vi "VI Linearisierung v2.vi"() -> ()   [LabVIEW 2020, in "Linearisierung v2.lvlib"] (continued)
                # "running erst setzen, wenn der Gasteiler bereits aus Beenden raus ist ,\nsonst triggert er im Timeout schon wieder ... !!!"
                n1604 = case shown="Kein Fehler" w2827 {
                  frame No Error {
                    n1605 = call "FGV SpanEinstellungen.vi"("Aktion"=Aktion_FGV_SpanEinstellungen."lesen") -> ("automatisch out"=w2832:T20)  [unwired: 6 in, 4 out]
                    n1606 = call "FGV Daten Abholung uebergeben.vi"("Aktion"=Aktion_FGV_Daten_Abholung_uebergebenctl."lesen") -> ("Beendet"=w2830:bool)  [unwired: 10 in, 4 out]
                    n1607 = call "FGV Gasteiler.vi"("Aktionen"=Aktionen_FGV_Gasteiler_Daten."lesen") -> ("Aufzeichnung Start"=w2828:bool)  [unwired: 11 in, 7 out]
                    n1608 = case shown="True" w2832 {
                      tunnel: w2830 -> [_ _]
                      tunnel: w2828 -> [_ _]
                      frame False {
                        # "brauchen wir hier auch !"
                        n1609 = call "FGV Spans abarbeiten.vi"("running"=TRUE, "Aktion"=Aktion_FGV_Spans_abarbeiten."running") -> ()  [unwired: 4 in, 6 out]
                      }
                      frame True {
                        # "für Start und Next erst hier"
                        n1610 = call "FGV Spans abarbeiten.vi"("running"=TRUE, "Aktion"=Aktion_FGV_Spans_abarbeiten."running") -> ()  [unwired: 4 in, 6 out]
                      }
                    }
                  }
                  frame Error {
                  }
                }
              }
              frame #5 {
                w2838 = T1 FALSE ("EPA Filename override")
                # "#LinV2_auto_singleSave"
                # "#RickQuickTest_Features"
                n1611 = call "FGV SpanEinstellungen.vi"("Aktion"=Aktion_FGV_SpanEinstellungen."lesen") -> ("Punkte umkehren und PDF Optionen Cluster"=w2840:T109)  [unwired: 6 in, 4 out]
                n1612 = Unbundle By Name(w2840) -> ("PDF Optionen.Graphik für Messwerte"=w2839:bool)
                n1613 = case shown="True" w2839 {
                  frame False {
                  }
                  frame True {
                    n1614 = call "LIN Graph.vi"() -> ()  [unwired: 12 in]
                  }
                }
                n1615 = local write "EPA Filename override"(w2838) -> ()
                n1616 = local write "LIN Filename override"(w2838) -> ()
              }
            }
          }
        }
        n1617 = local write "STARTEN"(w2640) -> ()
      }
      event Value Change {
        # "#Option10xSpanAuto"
        n1618 = event-data() -> ()  [unwired: 1 in, 1 out]
        n1619 = call "FGV Stoerungen sammeln und auswerten.vi"("Aktion"=Aktion_FGV_Stoerungen_sammeln_und_auswerten."lesen") -> ("Error"=w2848:bool)  [unwired: 12 in, 6 out]
        n1620 = disable-structure shown="Aktiviert" {
          frame Disabled {
            n1621 = call "FGV Spans abarbeiten.vi"("Aktion"=Aktion_FGV_Spans_abarbeiten."idle") -> ("error out"=w2862:errorcluster)  [unwired: 5 in, 5 out]
            n1622 = call "FGV SPAN Verriegelung.vi"("aktion"=Aktion_FGV_SPAN_Verriegelung."unlock", "error in (no error)"=w2862) -> ("error out"=w2861:errorcluster)  [unwired: 7 in, 2 out]
            n1623 = call "FGV Post Processing.vi"("Aktion"=Aktion_FGV_Post_Processing."reset", "error in (no error)"=w2861) -> ()  [unwired: 6 in, 4 out]
          }
          frame Enabled {
            # "#ALIN_Cancel_Save"
            n1624 = control-ref of="Speichern LIN"() -> (w2872:refnum<vi>)
            n1625 = call "FGV Spans abarbeiten.vi"("Aktion"=Aktion_FGV_Spans_abarbeiten."lesen") -> ("active SPAN Idx out"=w2868:i32)  [unwired: 5 in, 5 out]
            n1626 = call "FGV SpanEinstellungen.vi"("Aktion"=Aktion_FGV_SpanEinstellungen."lesen") -> ("SpanInletClusterArray out"=w2869:T19[])  [unwired: 6 in, 4 out]
            n1627 = call "get first active SPAN.vi"("SpanInletClusterArray in"=w2869) -> ("Index first active SPAN"=w2867:i32, "SpanInletClusterArray out"=w2865:T19[])  [unwired: 8 in, 1 out]
            n1628 = Greater?(x=w2868, y=w2867) -> (0:w2866:bool)
            n1629 = case shown="False" w2866 {
              tunnel: w2872 -> [_ w2883]
              tunnel: w2865 -> [_ w2880]
              frame False {
                # "nothing to save ..."
                n1630 = call "FGV Spans abarbeiten.vi"("Aktion"=Aktion_FGV_Spans_abarbeiten."idle") -> ("error out"=w2875:errorcluster)  [unwired: 5 in, 5 out]
                n1631 = call "FGV SPAN Verriegelung.vi"("aktion"=Aktion_FGV_SPAN_Verriegelung."unlock", "error in (no error)"=w2875) -> ("error out"=w2874:errorcluster)  [unwired: 7 in, 2 out]
                n1632 = call "FGV Post Processing.vi"("Aktion"=Aktion_FGV_Post_Processing."reset", "error in (no error)"=w2874) -> ()  [unwired: 6 in, 4 out]
              }
              frame True {
                n1633 = call "FGV Spans abarbeiten.vi"("Aktion"=Aktion_FGV_Spans_abarbeiten."abort") -> ("error out"=w2879:errorcluster)  [unwired: 5 in, 5 out]
                n1634 = call "FGV Post Processing.vi"("Aktion"=Aktion_FGV_Post_Processing."abort", "error in (no error)"=w2879, "SpanInletClusterArray in"=w2880) -> ("error out"=w2878:errorcluster)  [unwired: 5 in, 3 out]
                n1635 = call "FGV Spans abarbeiten.vi"("running"=FALSE, "Aktion"=Aktion_FGV_Spans_abarbeiten."running", "error in (no error)"=w2878) -> ("error out"=w2884:errorcluster)  [unwired: 3 in, 5 out]
                n1636 = property on="Eigenschaftsknoten" class="Bool. (strikt)"(reference=w2883, error in=w2884, "Val(Sgnl)"=T4 TRUE ("Wert (signalisierend)")) -> (error out=w2887:errorcluster)  [unwired: 1 out]
                n1637 = call <vilib>:"Clear Errors.vi"("error in (no error)"=w2887) -> ()  [unwired: 5 in, 2 out]
              }
            }
          }
        }
        n1638 = property class="Bool."(reference=w2843, "DisabledEnum"=T66."Disabled and Grayed Out" ("Deaktiviert")) -> (error out=w2845:errorcluster)  [unwired: 1 in, 1 out]
        n1639 = call "FGV Gasteiler.vi"("Aufzeichnung Start"=FALSE ("STARTEN"), "Aktionen"=Aktionen_FGV_Gasteiler_Daten."Aufzeichnung Start") -> ()  [unwired: 10 in, 8 out]
        n1640 = And(x=w2848, y="ABBRECHEN") -> (x .and. y?=w2850:T4)
        n1641 = call <vilib>:"Clear Errors.vi"("error in (no error)"=w2845) -> ()  [unwired: 5 in, 2 out]
        n1642 = call "FGV Stoerungen sammeln und auswerten.vi"("Abbrechen"=w2850, "Aktion"=Aktion_FGV_Stoerungen_sammeln_und_auswerten."abbrechen") -> ("error out"=w2853:errorcluster)  [unwired: 11 in, 6 out]
        n1643 = property on="FORTSETZEN" class="Bool."(error in=w2853, "Visible"=FALSE ("Sichtbar")) -> (error out=w2855:errorcluster)  [unwired: 1 in, 1 out]
        n1644 = call <vilib>:"Clear Errors.vi"("error in (no error)"=w2855) -> ("error out"=w2851:errorcluster)  [unwired: 5 in, 1 out]
        n1645 = call "FGV Stoerungen sammeln und auswerten.vi"("error in (no error)"=w2851, "Aktion"=Aktion_FGV_Stoerungen_sammeln_und_auswerten."reset error") -> ()  [unwired: 11 in, 7 out]
      }
      event "post processing": Value Change {
        # "#LIN_only_saved_Polynoms"
        n1646 = event-data() -> ("OldVal"=w2891:u16)  [unwired: 1 in, 5 out]
        n1647 = Greater Than 0?(x="post processing") -> (x > 0?=w2890:bool)
        n1648 = Decrement(x="post processing") -> (x-1=w2889:u16)
        n1649 = case shown="False" w2890 {
          tunnel: w2889 -> [_ w2910]
          tunnel: w2893 -> [_ w2911]
          tunnel: w2891 -> [w2897 w2907]
          frame False {
            n1650 = call "FGV SPAN Verriegelung.vi"("aktion"=Aktion_FGV_SPAN_Verriegelung."lesen") -> ("Flags Cluster"=w2900:T188)  [unwired: 8 in, 2 out]
            n1651 = local write "post processing"(w2897) -> ()
            n1652 = Unbundle By Name(w2900) -> ("Postprocessing PDF"=w2898:bool)
            n1653 = case shown="True" w2898 {
              frame False {
              }
              frame True {
                n1654 = local write "post processing PDFs"(T4 FALSE ("post processing PDFs")) -> ()
                n1655 = call "FGV SPAN Verriegelung.vi"("aktion"=Aktion_FGV_SPAN_Verriegelung."Reset Postprocessing PDF") -> ()  [unwired: 8 in, 3 out]
              }
            }
          }
          frame True {
            n1656 = Decrement(x=w2907) -> (x-1=w2906:u16)
            n1657 = call "FGV Post Processing.vi"("Aktion"=Aktion_FGV_Post_Processing."lesen") -> ("filenemas Cluster Array"=w2917:T211, "Index active SPANs"=w2909:i32[])  [unwired: 7 in, 2 out]
            n1658 = call "FGV SPAN Verriegelung.vi"("aktion"=Aktion_FGV_SPAN_Verriegelung."lesen") -> ("Flags Cluster"=w2905:T188)  [unwired: 8 in, 2 out]
            n1659 = Unbundle By Name(w2905) -> ("Postprocessing PDF"=w2903:bool)
            n1660 = Index Array(array=w2909, index=w2910) -> (element=w2913:i32)
            n1661 = Index Array(array=w2917, index=w2910) -> (element=w2916:T212)
            n1662 = Index Array(array=w2909, index=w2906) -> (element=w2908:i32)
            n1663 = Unbundle By Name(w2916) -> ("active SPAN Idx"=w2912:i32, "Pfad .LIN Datei"=w2915:T9)
            n1664 = Equal?(x=w2913, y=w2912) -> (x = y?=w2914:bool)
            n1665 = case shown="True" w2914 {
              tunnel: w2915 -> [_ w2954]
              tunnel: w2913 -> [w2924 w2930]
              tunnel: w2912 -> [w2922 _]
              tunnel: w2911 -> [_ w2952]
              tunnel: w2910 -> [_ w2946]
              tunnel: w2908 -> [_ w2942]
              tunnel: w2906 -> [_ w2934]
              tunnel: w2903 -> [_ w2927]
              tunnel: w2903 -> [_ w2926]
              frame False {
                n1666 = Number To Decimal String(number=w2924) -> (decimal integer string=w2923:string)  [unwired: 1 in]
                n1667 = Number To Decimal String(number=w2922) -> (decimal integer string=w2921:string)  [unwired: 1 in]
                n1668 = Concatenate Strings("internal Error: active SPAN ", w2923, " <> " ("String"), w2921) -> (w2919:string)
                n1669 = One Button Dialog(message=w2919) -> ()  [unwired: 1 in, 1 out]
              }
              frame True {
                w2945 = 0  # Component Idx
                # "#Lin_Load_Polynom_Question"
                n1670 = case shown="False" w2927 {
                  tunnel: w2942 -> [w2962 _]
                  tunnel: [w2961 _] -> w2935
                  tunnel: w2934 -> [w2960 _]
                  frame False {
                    n1671 = call "PostProcessing_LIN_speichern.vi"("Index active SPAN"=w2962, "reprocessing index for filname"=w2960) -> ("Fehler (Ausgang)"=w2961:errorcluster)  [unwired: 9 in]
                  }
                  frame True {
                  }
                }
                n1672 = call "Set SPAN Komponentauswahl in Protokolldaten.vi"("error in (no error)"=w2935, "index of element"=w2930) -> ("error out"=w2937:errorcluster, "original Lin-Polynom"=w2936:T119)  [unwired: 8 in]
                n1673 = Bundle("Index active SPAN"=w2930, "Component Idx"=w2945, w2946) -> (w2947:T213)  [unwired: 1 in]
                n1674 = call "FGV SpanEinstellungen.vi"("Aktion"=Aktion_FGV_SpanEinstellungen."lesen") -> ("SpanInletClusterArray out"=w2931:T19[])  [unwired: 6 in, 4 out]
                n1675 = call "LinDaten speichern und laden.vi"("Aktion"=enum16{"speichern", "laden"}."speichern", "error in (no error)"=w2937) -> ("error out"=w2955:errorcluster, "LIN Protokoll Daten"=w2943:T119, "Setup Daten-Cluster"=w2940:T204, "Settings Cluster"=w2941:T206)  [unwired: 3 in, 3 out]
                n1676 = Index Array(array=w2931, index=w2930) -> (element=w2933:T19)
                n1677 = Unbundle By Name(w2943) -> ("Messgerät"=w2944:string)
                n1678 = Unbundle By Name(w2933) -> ("Max Fehler"=w2928:sgl)
                n1679 = call "LinDaten speichern und laden.vi"("Aktion"=enum16{"speichern", "laden"}."laden", "error in (no error)"=w2955, "Analysator"=w2944, "selected path"=w2954) -> ("error out"=w2957:errorcluster, "LIN Protokoll Daten"=w2948:T119, "MessDaten Array"=w2949:string[][][], "Ident Cluster"=w2958:T205, "Setup Daten-Cluster"=w2938:T204, "Settings Cluster"=w2939:T206)  [unwired: 1 in, 1 out]
                n1680 = Bundle By Name(cluster=w2948, "F_max gefordert (%)"=w2928) -> (w2929:T119)
                n1681 = call "LIN Laden Errors.vi"("Fehler (Eingang, kein Fehler)"=w2957, "Ident Cluster"=w2958) -> ("Error orccured"=w2953:bool, "LIN Loading Error Description Array"=w2951:T207, "LIN Loading Errors Array"=w2950:string[])  [unwired: 5 in, 2 out]
                n1682 = case shown="False" w2953 {
                  tunnel: w2952 -> [_ w2993]
                  tunnel: w2951 -> [_ _]
                  tunnel: w2950 -> [_ w2986]
                  tunnel: w2949 -> [w2980 _]
                  tunnel: w2929 -> [w2970 _]
                  tunnel: w2947 -> [w2976 _]
                  tunnel: w2941 -> [w2974 _]
                  tunnel: w2940 -> [w2973 _]
                  tunnel: w2939 -> [w2972 _]
                  tunnel: w2938 -> [w2971 _]
                  tunnel: w2936 -> [_ w2987]
                  tunnel: w2930 -> [w2966 _]
                  tunnel: w2926 -> [w2963 _]
                  frame False {
                    n1683 = call "Lin Daten aufarbeiten.vi"("Lin-Polynom"=w2970, "Aktionen"=Aktion_Lin_Daten_aufarbeiten."Protkolldaten") -> ("Lin-Polynom"=w2968:T119, "error out"=w2969:errorcluster)  [unwired: 15 in, 9 out]
                    n1684 = call "Lin Daten aufarbeiten.vi"("error in (no error)"=w2969, "TabellenArray"=w2980, "Aktionen"=Aktion_Lin_Daten_aufarbeiten."Nachbehandlung laden") -> ("error out"=w2967:errorcluster)  [unwired: 14 in, 10 out]
                    n1685 = call "LIN Laden Polynom setzen.vi"("Span Iindex"=w2966, "Settings Cluster old"=w2974, "Setup Daten-Cluster old"=w2973, "error in (no error)"=w2967, "LIN Protokoll Daten"=w2968, "Setup Daten-Cluster new"=w2971, "Settings Cluster new"=w2972) -> ("error out"=w2965:errorcluster)  [unwired: 4 in]
                    n1686 = call "FGV Post Processing.vi"("Aktion"=Aktion_FGV_Post_Processing."active", "error in (no error)"=w2965, "active Index Cluster in"=w2976) -> ("error out"=w2977:errorcluster)  [unwired: 5 in, 3 out]
                    n1687 = property on="Gasnummer Generieren" class="DigWert (strikt)"(error in=w2977, "Val(Sgnl)"=T49 1 ("Wert (signalisierend)")) -> (error out=w2964:errorcluster)  [unwired: 1 in, 1 out]
                    n1688 = case shown="True" w2963 {
                      tunnel: w2964 -> [_ w2982]
                      frame False {
                      }
                      frame True {
                        n1689 = property on="Speichern LIN" class="Bool. (strikt)"(error in=w2982, "Val(Sgnl)"=T4 TRUE ("Wert (signalisierend)")) -> (error out=w2984:errorcluster)  [unwired: 1 in, 1 out]
                        n1690 = call <vilib>:"Clear Errors.vi"("error in (no error)"=w2984) -> ()  [unwired: 5 in, 2 out]
                      }
                    }
                  }
                  frame True {
                    # "reset"
                    n1691 = call "Lin Daten aufarbeiten.vi"("Lin-Polynom"=w2987, "Aktionen"=Aktion_Lin_Daten_aufarbeiten."Protkolldaten") -> ()  [unwired: 15 in, 11 out]
                    n1692 = call "Texte in VIs uebersetzen.vi"("Sprachliste"=w2993, "String-Array zum Übersetzen"=w2986, "String zum Übersetzen"="Loading LIN Date does not fit actual Setup!") -> ("String-Array zum Übersetzen"=w2985:string[], "String zum Übersetzen"=w2994:string)  [unwired: 8 in, 3 out]
                    n1693 = call <vilib>:"1D String Array to Delimited String.vi"("delimiter"=",", "string array"=w2985) -> ("delimited string"=w2989:string)  [unwired: 9 in]
                    n1694 = Concatenate Strings(w2994, " - " ("String"), w2989) -> (w2992:string)
                    n1695 = One Button Dialog(message=w2992) -> ()  [unwired: 1 in, 1 out]
                  }
                }
              }
            }
          }
        }
      }
      event Value Change {
        n1696 = event-data() -> ()  [unwired: 1 in, 6 out]
        n1697 = call "FGV SPAN Verriegelung.vi"("aktion"=Aktion_FGV_SPAN_Verriegelung."lesen") -> ("Flags Cluster"=w2997:T188)  [unwired: 8 in, 2 out]
        n1698 = Unbundle By Name(w2997) -> ("Postprocessing PDF"=w2996:bool)
        n1699 = case shown="False" w2996 {
          tunnel: w2999 -> [w3004 _]
          frame False {
            n1700 = call "Texte in VIs uebersetzen.vi"("Sprachliste"=w3004, "String zum Übersetzen"="Alle PDF vom Postprocessing speichern?" ("Nachricht")) -> ("String zum Übersetzen"=w3010:string)  [unwired: 9 in, 4 out]
            n1701 = call "Texte in VIs uebersetzen.vi"("Sprachliste"=w3004, "String zum Übersetzen"="Ja" ("Text für T-Schaltfläche (\"OK\")")) -> ("String zum Übersetzen"=w3009:string)  [unwired: 9 in, 4 out]
            n1702 = call "Texte in VIs uebersetzen.vi"("Sprachliste"=w3004, "String zum Übersetzen"="Nein" ("Text für F-Schaltfläche (\"Abbrechen\")")) -> ("String zum Übersetzen"=w3008:string)  [unwired: 9 in, 4 out]
            n1703 = Two Button Dialog(message=w3010, 1:w3008, 2:w3009) -> (T button?=w3003:bool)
            n1704 = case shown="True" w3003 {
              frame False {
              }
              frame True {
                w3011 = FALSE
                # "#LinV2_auto_singleSave"
                # "letzte Änderung beim ersten Aufruf speichern\nruft signalisierend Postprocessing Span Auswahl auf ..."
                n1705 = local read "post processing"() -> (w3019:u16)
                n1706 = call "FGV Post Processing.vi"("Aktion"=Aktion_FGV_Post_Processing."lesen") -> ("Index active SPANs"=w3018:i32[])  [unwired: 7 in, 3 out]
                n1707 = Decrement(x=w3019) -> (x-1=w3012:u16)
                n1708 = Index Array(array=w3018, index=w3012) -> (element=w3020:i32)
                n1709 = call "PostProcessing_LIN_speichern.vi"("Index active SPAN"=w3020, "reprocessing index for filname"=w3012) -> ("Fehler (Ausgang)"=w3013:errorcluster)  [unwired: 9 in]
                n1710 = call "FGV SPAN Verriegelung.vi"("aktion"=Aktion_FGV_SPAN_Verriegelung."Set Postprocessing PDF", "error in (no error)"=w3013) -> ("error out"=w3016:errorcluster)  [unwired: 7 in, 2 out]
                n1711 = local write "EPA Filename override"(w3011) -> ()
                n1712 = local write "LIN Filename override"(w3011) -> ()
                n1713 = call "FGV Post Processing.vi"("Aktion"=Aktion_FGV_Post_Processing."first", "error in (no error)"=w3016) -> ()  [unwired: 6 in, 4 out]
              }
            }
          }
          frame True {
            # "läuft schon"
            n1714 = local write "post processing PDFs"(T4 FALSE ("post processing PDFs")) -> ()
          }
        }
      }
      event Value Change {
        n1715 = event-data() -> ()  [unwired: 1 in, 1 out]
        n1716 = local write "post processing done"(T4 FALSE ("post processing done")) -> ()
        n1717 = call "Texte in VIs uebersetzen.vi"("Sprachliste"=w3024, "String zum Übersetzen"="Fertig mit Postprocessing?\nFreigabe löscht die gesammelten Daten!" ("Nachricht")) -> ("String zum Übersetzen"=w3026:string)  [unwired: 9 in, 4 out]
        n1718 = call "Texte in VIs uebersetzen.vi"("Sprachliste"=w3024, "String zum Übersetzen"="Ja" ("Text für T-Schaltfläche (\"OK\")")) -> ("String zum Übersetzen"=w3027:string)  [unwired: 9 in, 4 out]
        n1719 = call "Texte in VIs uebersetzen.vi"("Sprachliste"=w3024, "String zum Übersetzen"="Nein" ("Text für F-Schaltfläche (\"Abbrechen\")")) -> ("String zum Übersetzen"=w3028:string)  [unwired: 9 in, 4 out]
        n1720 = Two Button Dialog(message=w3026, 1:w3028, 2:w3027) -> (T button?=w3025:bool)
        n1721 = case shown="True" w3025 {
          frame False {
          }
          frame True {
            n1722 = call "FGV Post Processing.vi"("Aktion"=Aktion_FGV_Post_Processing."reset") -> ("error out"=w3034:errorcluster)  [unwired: 7 in, 3 out]
            n1723 = call "FGV SPAN Verriegelung.vi"("aktion"=Aktion_FGV_SPAN_Verriegelung."unlock", "error in (no error)"=w3034) -> ()  [unwired: 7 in, 3 out]
          }
        }
      }
      event Value Change {
        # "#LIN_only_saved_Polynoms"
        # "#PDF_manu_MG"
        n1724 = event-data() -> ()  [unwired: 1 in, 1 out]
        n1725 = call "Komponentenausgabe.vi"() -> ("Gaskomponente"=w3051:T7)  [unwired: 8 in, 3 out]
        n1726 = local read "Gasnummer LIN"() -> (w3042:T49)
        n1727 = call "Lin Daten aufarbeiten.vi"("Index (Seite)"=w3051, "Polynom-Ordnung"="Polynom-Ordnung", "Aktionen"=Aktion_Lin_Daten_aufarbeiten."Lin auswerten") -> ("Index (Seite) out"=w3044:i32, "error out"=w3053:errorcluster)  [unwired: 14 in, 9 out]
        n1728 = call "aktueller SPAN und Komponent Index.vi"() -> ("akt SPAN out"=w3039:i32)  [unwired: 7 in, 4 out]
        n1729 = Decrement(x=w3042) -> (x-1=w3038:T49)
        n1730 = Bundle("akt SPAN out"=w3039, w3038) -> (w3037:cluster{"akt SPAN out":i32, T49})  [unwired: 1 in]
        n1731 = call "Lin Daten aufarbeiten.vi"("Index (Seite)"=w3044, "error in (no error)"=w3053, "Aktionen"=Aktion_Lin_Daten_aufarbeiten."lesen") -> ("Eingabetabelle"=w3052:T54, "Lin-Polynom"=w3049:T119)  [unwired: 14 in, 9 out]
        n1732 = call "LIN Polynom Ordnung je Komponente für Protokoll.vi"("Aktion"=Aktion_LIN_Polynom_Ordnung_je_Komponente_für_Protokoll."schreiben viewonly", "Polynom-Ordnung view only"="Polynom-Ordnung", "Index in"=w3037) -> ()  [unwired: 2 in, 7 out]
        n1733 = Unbundle By Name(w3049) -> ("Polynomkoeff."=w3048:dbl[])
        n1734 = call "LinTabelle zusammenbauen.vi"("Eingabetabelle"=w3052) -> ("XY-Graph"=w3050:cluster{dbl[], dbl[]}[], "LIN Ausgabetabelle"=w3056:string[][])  [unwired: 7 in, 2 out]
        n1735 = local write "LIN Ausgabetabelle"(w3056) -> ()
        n1736 = local write "XY-Graph LIN"(w3050) -> ()
        n1737 = Array To Cluster(array=w3048) -> (cluster=→"LIN Polynomkoeffizienten":T185)
      }
      event Value Change {
        n1738 = event-data() -> ()  [unwired: 1 in, 1 out]
        n1739 = stacked-sequence {
          seq-local: [_ w3072 _ _] -> [_ _ w3095 _]
          seq-local: [_ w3071 _ _] -> [_ _ w3094 _]
          seq-local: [_ w3070 _ _] -> [_ _ w3096 _]
          seq-local: [_ _ w3088 _] -> [_ _ _ w3115]
          tunnel: w3060 -> [_ _ w3087 w3118]
          frame #0 {
            # "#LIN_only_saved_Polynoms"
            n1740 = call "Lin Daten aufarbeiten.vi"("Aktionen"=Aktion_Lin_Daten_aufarbeiten."lesen") -> ("Lin-Polynom"=w3068:T119)  [unwired: 16 in, 10 out]
            n1741 = Unbundle By Name(w3068) -> ("Polynomkoeff."=w3064:dbl[])
            n1742 = call "Komponentenausgabe.vi"() -> ("Gaskomponente"=w3061:T7)  [unwired: 8 in, 3 out]
            n1743 = call "Polynom Daten speichern.vi"("Aktionen"=Aktionen_Polynom_Daten_speichern."schreiben", "Einzelnes Polynom"=w3064, "Komponente"=w3061) -> ("Aktiv"=w3067:bool[])  [unwired: 3 in, 5 out]
            n1744 = call "Polynom Daten speichern.vi"("Aktionen"=Aktionen_Polynom_Daten_speichern."aktivieren", "Aktiv"=w3067, "Komponente"=w3061) -> ("Aktiv"=w3062:bool[])  [unwired: 3 in, 5 out]
            n1745 = call "Polynom Daten speichern.vi"("Aktionen"=Aktionen_Polynom_Daten_speichern."speichern", "Aktiv"=w3062) -> ()  [unwired: 4 in, 6 out]
          }
          frame #1 {
            # "#LIN_only_saved_Polynoms\nIstwerte mit neuem Polynom neu berechnen und anzeigen.\nEinstellungen speichern für Protokoll,\nin .LIN ebenfalls und wieder laden !\naktuell: aktuell + ---, 1...4\nautom.: automatisch + keine, 1...4\nmanuell: manuell + keine, 1...4\nraw: manuell + keine"
            n1746 = call "Komponentenausgabe.vi"() -> ("error out"=w3085:errorcluster, "Gaskomponente"=w3084:T7)  [unwired: 8 in, 2 out]
            n1747 = call "Lin Daten aufarbeiten.vi"("Index (Seite)"=w3084, "error in (no error)"=w3085, "Aktionen"=Aktion_Lin_Daten_aufarbeiten."LIN übernehmen") -> ("Index (Seite) out"=w3074:i32, "error out"=w3075:errorcluster)  [unwired: 14 in, 9 out]
            n1748 = call "aktueller SPAN und Komponent Index.vi"() -> ("akt SPAN out"=w3072:i32, "SpanInletClusterArray out"=w3070:T19[])  [unwired: 7 in, 3 out]
            n1749 = call "Lin Daten aufarbeiten.vi"("Index (Seite)"=w3074, "error in (no error)"=w3075, "Aktionen"=Aktion_Lin_Daten_aufarbeiten."lesen") -> ("Eingabetabelle"=w3077:T54, "error out"=w3076:errorcluster)  [unwired: 14 in, 9 out]
            n1750 = local read "Polynom-Ordnung"() -> (w3079:T55)
            n1751 = local read "Gasnummer LIN"() -> (w3086:T49)
            n1752 = call "LinTabelle zusammenbauen.vi"("error in (no error)"=w3076, "Eingabetabelle"=w3077) -> ("error out"=w3081:errorcluster, "LIN Ausgabetabelle"=w3082:string[][])  [unwired: 6 in, 2 out]
            n1753 = Decrement(x=w3086) -> (x-1=w3071:T49)
            n1754 = Bundle("akt SPAN out"=w3072, w3071) -> (w3073:cluster{"akt SPAN out":i32, T49})  [unwired: 1 in]
            n1755 = call "LIN Polynom Ordnung je Komponente für Protokoll.vi"("Aktion"=Aktion_LIN_Polynom_Ordnung_je_Komponente_für_Protokoll."schreiben", "error in (no error)"=w3081, "Index in"=w3073, "Polynom-Ordnung"=w3079) -> ()  [unwired: 1 in, 7 out]
            n1756 = local write "LIN Ausgabetabelle"(w3082) -> ()
          }
          frame #2 {
            # "Changes Flag setzen (vor der nächsten postprocess Auswahl dann .LIN speichern)\nKontrollieren ob in eine der Komponenten eines anderen SPAN die selbe ist,\ndann Warnung das kontrolliert werden soll, weil das dann automatisch auch so gerechnet wird beim Speichern wenn Done.\nBeim Laden der .LIN wird ein ungleiches Polynom erkannt und der Istwert neu berechnet (mit Hinweis) \nund die Polynomauswahl auf \"automatisch\" gesetzt."
            n1757 = call "get SPANs for same components in postprocessing.vi"("active Component Index"=w3094, "active SPAN Idx"=w3095, "SpanInletClusterArray in"=w3096) -> ("error out"=w3091:errorcluster, "active SPAN Idx out"=w3093:i32, "SPAN Index Array mit gleicher Komponente"=w3090:i32[], "found"=w3092:bool)  [unwired: 2 in, 3 out]
            n1758 = call "LIN Polynom Ordnung oder Aktiv Changes für Postprocessing.vi"("Aktion"=Aktion_LIN_Polynom_Ordnung_ode_Aktiv_Changes_für_Postprocessing."schreiben", "error in (no error)"=w3091, "active SPAN Idx"=w3093, "Changes"=TRUE) -> ()  [unwired: 4 in, 4 out]
            n1759 = case shown="True" w3092 {
              tunnel: w3090 -> [_ w3103]
              tunnel: ["" w3099] -> w3088
              tunnel: w3087 -> [_ w3107]
              frame False {
              }
              frame True {
                w3104 = "\r"
                n1760 = for {
                  tunnel: w3103 -> [w3114] mode=indexing
                  tunnel: "SPAN" -> [w3113]
                  shift-right: [w3110] -> w3100
                  shift-left: "" -> [w3109]
                  n1761 = Increment(x=w3114) -> (x+1=w3108:i32)
                  n1762 = Number To Decimal String(number=w3108) -> (decimal integer string=w3112:string)  [unwired: 1 in]
                  n1763 = call <vilib>:"Space Constant.vi"() -> ("String"=w3111:string)
                  n1764 = Concatenate Strings(w3109, w3113, w3112, w3111) -> (w3110:string)
                }
                n1765 = call "Texte in VIs uebersetzen.vi"("Sprachliste"=w3107, "String zum Übersetzen"="Polynom wird auch in anderen SPAN Komponenten verwendet !") -> ("String zum Übersetzen"=w3105:string)  [unwired: 9 in, 4 out]
                n1766 = Concatenate Strings(w3104, w3105, w3104, w3100) -> (w3099:string)
              }
            }
          }
          frame #3 {
            n1767 = call "Texte in VIs uebersetzen.vi"("Sprachliste"=w3118, "String zum Übersetzen"="Neues Polynom gespeichert!" ("Nachricht")) -> ("String zum Übersetzen"=w3119:string)  [unwired: 9 in, 4 out]
            n1768 = Concatenate Strings(w3119, w3115) -> (w3116:string)
            n1769 = One Button Dialog(message=w3116) -> ()  [unwired: 1 in, 1 out]
          }
        }
      }
      event Value Change {
        n1770 = event-data() -> ()  [unwired: 1 in, 1 out]
        n1771 = control-ref of="FORTSETZEN"() -> (w3121:refnum<vi>)
        n1772 = call "Fortsetzen Reset.vi"("FORTSETZEN"="FORTSETZEN", "Referenz Boolesch (Eingang)"=w3121) -> ()  [unwired: 10 in]
        n1773 = property class="Bool."(reference=w3122, "DisabledEnum"=T66."Enabled" ("Deaktiviert")) -> (error out=w3124:errorcluster)  [unwired: 1 in, 1 out]
        n1774 = call <vilib>:"Clear Errors.vi"("error in (no error)"=w3124) -> ()  [unwired: 5 in, 2 out]
      }
      event Value Change {
        n1775 = event-data() -> ("OldVal"=w3138:T54, "NewVal"=w3137:T54)  [unwired: 1 in]
        n1776 = call "Nur Zahlen durchlassen.vi"("alte Tabelle"=w3138, "neue Tabelle"=w3137) -> ("neue Tabelle"=w3140:string[][])  [unwired: 12 in, 1 out]
        n1777 = call "Tabelle auffeullen.vi"("Neue Tabelle"=w3140) -> ("Tabelle"=w3139:string[][])  [unwired: 10 in]
        n1778 = call "Komponentenausgabe.vi"() -> ("Gaskomponente"=w3131:T7)  [unwired: 8 in, 3 out]
        n1779 = call "Lin Daten aufarbeiten.vi"("Eingabetabelle"=w3139, "Index (Seite)"=w3131, "Aktionen"=Aktion_Lin_Daten_aufarbeiten."Tabelle schreiben") -> ("Index (Seite) out"=w3130:i32, "error out"=w3135:errorcluster)  [unwired: 14 in, 9 out]
        n1780 = call "Lin Daten aufarbeiten.vi"("Index (Seite)"=w3130, "error in (no error)"=w3135, "Polynom-Ordnung"=Auswahl_Polynom_Ordnung."actual", "Aktionen"=Aktion_Lin_Daten_aufarbeiten."Lin auswerten") -> ("Index (Seite) out"=w3132:i32, "error out"=w3136:errorcluster)  [unwired: 13 in, 9 out]
        n1781 = call "Lin Daten aufarbeiten.vi"("Index (Seite)"=w3132, "error in (no error)"=w3136, "Aktionen"=Aktion_Lin_Daten_aufarbeiten."lesen") -> ("Eingabetabelle"=w3142:T54, "error out"=w3144:errorcluster)  [unwired: 14 in, 9 out]
        n1782 = call "AusgabeTabelle zusammenbauen.vi"("error in (no error)"=w3144, "Eingabetabelle"=w3142) -> ("Eingabetabelle behandelt"=w3141:string[][], "Ausgabetabelle"=w3143:T53)  [unwired: 7 in, 1 out]
        n1783 = local write "Ausgabetabelle"(w3143) -> ()
        n1784 = local write "Eingabetabelle"(w3141) -> ()
      }
      event "TCP Verbindung aktiv", "IP 1", "IP 2", "IP 3", "IP 4", "Port": Value Change {
        w3166 = "." ("String")
        n1785 = event-data() -> ()  [unwired: 1 in, 6 out]
        n1786 = Number To Decimal String(number="IP 1") -> (decimal integer string=w3167:string)  [unwired: 1 in]
        n1787 = Number To Decimal String(number="IP 2") -> (decimal integer string=w3165:string)  [unwired: 1 in]
        n1788 = Number To Decimal String(number="IP 3") -> (decimal integer string=w3164:string)  [unwired: 1 in]
        n1789 = Number To Decimal String(number="IP 4") -> (decimal integer string=w3163:string)  [unwired: 1 in]
        n1790 = Boolean To (0,1)(Boolean="TCP Verbindung aktiv") -> (0, 1=w3153:i16)
        n1791 = Concatenate Strings(w3167, w3166, w3165, w3166, w3164, w3166, w3163) -> (w3162:string)
        n1792 = local write "Registerkarte"(w3153) -> ()
        n1793 = Bundle("TCP Verbindung aktiv"="TCP Verbindung aktiv", w3162, "Port"="Port") -> (w3161:T214)  [unwired: 1 in]
        n1794 = call "FGV Gasteiler.vi"("TCP"=w3161, "Aktionen"=Aktionen_FGV_Gasteiler_Daten."TCP") -> ("Serielle Parameter"=w3160:T129)  [unwired: 10 in, 7 out]
        n1795 = call "FGV Gasteiler.vi"("Serielle Parameter"=w3160, "Aktionen"=Aktionen_FGV_Gasteiler_Daten."speichern") -> ()  [unwired: 10 in, 8 out]
      }
      event Value Change {
        w3184 = TRUE  # manuelle Anforderung
        w3183 = TRUE  # show Message
        w3193 = FALSE  # auto Scan
        # "#Option10xSpanAuto"
        n1796 = event-data() -> ("CtlRef"=w3195:refnum<vi>)  [unwired: 1 in]
        n1797 = Search 1D Array(1D array=w3196, element=w3195) -> (index of element=w3169:i32)  [unwired: 1 in]
        n1798 = control-ref of="Anforderung"() -> (w3181:refnum<vi>)
        n1799 = Index Array(array=w3189, index=w3169) -> (element=w3194:refnum<vi>)
        n1800 = Bundle By Name(cluster=T152 {"Stufen Tabelle Array"=[], "auto Scan Points"=[], "Punkte umkehren"=[], "Parameterkontrolle Array"=[], "Eingabetabelle"=refnum, "Ausgabetabelle"=refnum, "Anforderung"=refnum, "Status Str Referenz"=refnum, "Prüfgasnamen Array"=[]} ("Referenzen Cluster"), "Stufen Tabelle Array"=w3190, "auto Scan Points"=w3189, "Punkte umkehren"=w3188, "Parameterkontrolle Array"=w3187, "Eingabetabelle"=w3186, "Ausgabetabelle"=w3185, "Anforderung"=w3181, "Prüfgasnamen Array"=w3171) -> (w3175:T152)
        n1801 = property class="Bool. (strikt)"(reference=w3194, "Value"=w3193) -> (error out=w3192:errorcluster)  [unwired: 1 in, 1 out]
        n1802 = local read "Gasteiler Span Eingänge"() -> (w3172:u16)
        n1803 = call "FGV SpanEinstellungen.vi"("Aktion"=Aktion_FGV_SpanEinstellungen."lesen") -> ("SpanInletClusterArray out"=w3178:T19[])  [unwired: 6 in, 4 out]
        n1804 = call "set Tables Flag from SPANIdx.vi"("SPAN Idx"=w3169) -> ("set Tables"=w3170:bool)  [unwired: 10 in]
        n1805 = Bundle("manuelle Anforderung"=w3184, "show Message"=w3183, "set Tables"=w3170, "set Tables"=w3170) -> (w3180:T215)  [unwired: 1 in]
        n1806 = call <vilib>:"Clear Errors.vi"("error in (no error)"=w3192) -> ()  [unwired: 5 in, 2 out]
        n1807 = call "SPAN GD Test alle Formeln.vi"("GD Span Eingänge"=w3172, "Sprachliste"=w3174, "manueller SPAN Index in"=w3169, "Referenzen Cluster"=w3175, "SpanInletClusterArray in"=w3178) -> ("error out"=w3176:errorcluster, "SpanInletClusterArray out"=w3177:T19[], "GD LNI Cluster"=w3173:T208)  [unwired: 3 in, 1 out]
        n1808 = case shown="Kein Fehler" w3176 {
          tunnel: w3174 -> [w3209 _]
          tunnel: w3180 -> [w3208 _]
          tunnel: w3175 -> [w3207 _]
          tunnel: w3169 -> [w3206 _]
          tunnel: w3177 -> [w3205 _]
          tunnel: w3173 -> [w3204 _]
          tunnel: w3170 -> [w3201 _]
          tunnel: w3168 -> [w3199 _]
          frame No Error {
            # "#STB_keep"
            n1809 = call "SPAN Stufen abfragen Gasteiler alle Komponenten.vi"("GD LNI Cluster"=w3204, "Sprachliste"=w3209, "Boolsche Flags Cluster"=w3208, "Referenzen Cluster"=w3207, "SPAN Index in"=w3206, "SpanInletClusterArray in"=w3205) -> ("error out"=w3200:errorcluster, "Component Index out"=w3203:i32, "SPAN Index out"=w3202:i32)  [unwired: 1 in, 2 out]
            n1810 = call "Set SPAN for Gasnumber Settings.vi"("set Tables"=w3201, "error in (no error)"=w3200, "Component Index"=w3203, "SPNA index"=w3202, "Digital (Eingang)"=w3199) -> ()  [unwired: 6 in, 1 out]
          }
          frame Error {
          }
        }
      }
      event Value Change {
        # "#HovaCALErrors"
        n1811 = event-data() -> ()  [unwired: 1 in, 1 out]
        n1812 = disable-structure shown="Deaktiviert" {
          frame Disabled {
            n1813 = call "FGV Passwortlevel.vi"("FGV Passwort Aktion"=FGV_Passwort_Aktion."prüfen", "geforderter Level"=i16 8) -> ()  [unwired: 2 in, 8 out]
          }
          frame Enabled {
          }
        }
        n1814 = call "FGV Stoerungen sammeln und auswerten.vi"("Errors"=T156 {"Störung Kommunikation"=FALSE, "Pressure carrier gas"=FALSE, "Pressure diluted gas"=FALSE, "Outlet Pressure"=FALSE, "SNOX before SAIR"=FALSE, "Störung Gasteiler"=FALSE} ("Eingangs-Cluster"), "Aktion"=Aktion_FGV_Stoerungen_sammeln_und_auswerten."error") -> ("error out"=w3215:errorcluster)  [unwired: 11 in, 6 out]
        n1815 = call "FGV Stoerungen sammeln und auswerten.vi"("error in (no error)"=w3215, "Aktion"=Aktion_FGV_Stoerungen_sammeln_und_auswerten."reset error") -> ("Errors"=w3214:T156, "error out"=w3211:errorcluster)  [unwired: 11 in, 5 out]
        n1816 = Unbundle By Name(w3214) -> ("Störung Kommunikation"=w3213:bool)
        n1817 = local write "Error"(T17 {"Pressure carrier gas"=FALSE, "Pressure diluted gas"=FALSE, "Outlet Pressure"=FALSE, "SNOX before SAIR"=FALSE} ("Error")) -> ()
        n1818 = call "FGV Gasteiler.vi"("Anforderung"="Anforderung", "error in (no error)"=w3211, "Aktionen"=Aktionen_FGV_Gasteiler_Daten."Anforderung") -> ()  [unwired: 9 in, 8 out]
        n1819 = case shown="False" "Anforderung" {
          frame False {
            n1820 = local write "Gasteilerstatus"("" ("Gasteilerstatus")) -> ()
          }
          frame True {
          }
        }
        n1821 = local write "Störung Kommunikation"(w3213) -> ()
      }
      event Value Change {
        w3246 = T15 5 items=["LNI", "Analog-Display", "AVL GDU", "Horiba GDC", "HovaCal", "Horiba SGD 710C"] ("y")
        w3247 = T15 4 items=["LNI", "Analog-Display", "AVL GDU", "Horiba GDC", "HovaCal", "Horiba SGD 710C"] ("y")
        # "#Option10xSpanAutoOption10xSpanAuto"
        n1822 = event-data() -> ("CtlRef"=w3250:refnum<vi>, "NewVal"=w3252:T27, "OldVal"=w3226:T27)  [unwired: 1 in]
        n1823 = call "FGV Gasteiler.vi"("Aktionen"=Aktionen_FGV_Gasteiler_Daten."lesen") -> ("Gasteiler Type"=w3245:T15, "Anforderung"=w3228:bool)  [unwired: 11 in, 6 out]
        n1824 = control-ref of="Anforderung"() -> (w3236:refnum<vi>)
        n1825 = disable-structure shown="TestRun==FALSE, Standard" {
          disable-tunnel: [FALSE TRUE] -> w3239
          frame condition #0 {
          }
          frame condition #1 (active) {
          }
        }
        n1826 = local read "Gasteiler Span Eingänge"() -> (w3232:u16)
        n1827 = Bundle By Name(cluster=T152 {"Stufen Tabelle Array"=[], "auto Scan Points"=[], "Punkte umkehren"=[], "Parameterkontrolle Array"=[], "Eingabetabelle"=refnum, "Ausgabetabelle"=refnum, "Anforderung"=refnum, "Status Str Referenz"=refnum, "Prüfgasnamen Array"=[]} ("Referenzen Cluster"), "Stufen Tabelle Array"=w3238, "auto Scan Points"=w3235, "Punkte umkehren"=w3234, "Parameterkontrolle Array"=w3233, "Eingabetabelle"=w3230, "Ausgabetabelle"=w3229, "Anforderung"=w3236, "Prüfgasnamen Array"=w3231) -> (w3237:T152)
        n1828 = Equal?(x=w3245, y=w3247) -> (x = y?=w3240:bool)
        n1829 = Equal?(x=w3245, y=w3246) -> (x = y?=w3241:bool)
        n1830 = Compound Arithmetic op=OR ("Mehrfacharithmetik")(w3239, w3228, w3240, w3241) -> (w3249:bool)
        n1831 = case shown="True" w3249 {
          tunnel: w3252 -> [_ w3269]
          tunnel: w3226 -> [_ w3267]
          tunnel: w3250 -> [_ w3285]
          tunnel: w3238 -> [_ w3288]
          tunnel: w3233 -> [_ w3287]
          tunnel: w3235 -> [_ w3286]
          tunnel: w3242 -> [w3260 w3270]
          tunnel: w3241 -> [w3258 w3274]
          tunnel: w3240 -> [w3257 _]
          tunnel: w3239 -> [w3256 _]
          tunnel: w3237 -> [_ w3280]
          tunnel: w3228 -> [_ w3279]
          tunnel: w3232 -> [_ w3276]
          tunnel: w3231 -> [_ w3275]
          tunnel: w3230 -> [_ w3273]
          tunnel: w3229 -> [_ w3272]
          tunnel: w3227 -> [_ w3271]
          frame False {
            n1832 = Compound Arithmetic op=OR ("Mehrfacharithmetik")(w3256, w3257, w3258) -> (w3259:bool)
            n1833 = case shown="False" w3259 {
              tunnel: w3260 -> [w3262 _]
              frame False {
                n1834 = call "Texte in VIs uebersetzen.vi"("Sprachliste"=w3262, "String zum Übersetzen"="Keine Anforderung Gasteiler!" ("Status")) -> ("String zum Übersetzen"=w3261:string)  [unwired: 9 in, 4 out]
                n1835 = One Button Dialog(message=w3261) -> ()  [unwired: 1 in, 1 out]
              }
              frame True {
              }
            }
          }
          frame True {
            # "#LIN_GDStufen_Anzahl"
            n1836 = call "FGV SpanEinstellungen.vi"("Aktion"=Aktion_FGV_SpanEinstellungen."lesen") -> ("error out"=w3282:errorcluster, "automatisch out"=w3278:T20, "SpanInletClusterArray out"=w3264:T19[])  [unwired: 6 in, 2 out]
            n1837 = Search 1D Array(1D array=w3288, element=w3285) -> (index of element=w3265:i32)  [unwired: 1 in]
            n1838 = case shown="True" w3279 {
              tunnel: w3264 -> [w3290 w3300]
              tunnel: w3265 -> [_ w3299]
              tunnel: [w3289 w3298] -> w3283
              tunnel: w3282 -> [w3289 w3297]
              tunnel: [w3290 w3296] -> w3281
              tunnel: w3270 -> [_ w3295]
              tunnel: w3280 -> [_ w3294]
              tunnel: w3278 -> [_ w3293]
              tunnel: [_ w3292] -> w3277
              tunnel: w3276 -> [_ w3291]
              frame False {
              }
              frame True {
                n1839 = call "SPAN GD Test alle Formeln.vi"("GD Span Eingänge"=w3291, "Sprachliste"=w3295, "manueller SPAN Index in"=w3299, "error in (no error)"=w3297, "automatisch in"=w3293, "Referenzen Cluster"=w3294, "SpanInletClusterArray in"=w3300) -> ("error out"=w3298:errorcluster, "SpanInletClusterArray out"=w3296:T19[], "GD LNI Cluster"=w3292:T208)  [unwired: 1 in, 1 out]
              }
            }
            n1840 = call "Stufentabelle auf Anzahl Punkte begrenzen.vi"("SpanInletClusterArray in"=w3264, "index of element in"=w3265, "Stufen Tabelle in"=w3269) -> ("Stufen Tabelle out"=w3268:T27)  [unwired: 6 in, 2 out]
            n1841 = call "Stufentabelle auf Anzahl Punkte begrenzen.vi"("SpanInletClusterArray in"=w3264, "index of element in"=w3265, "Stufen Tabelle in"=w3267) -> ("Stufen Tabelle out"=w3266:T27)  [unwired: 6 in, 2 out]
            n1842 = case shown="Kein Fehler" w3283 {
              selector: w3283 -> [w3333 _]
              tunnel: w3287 -> [w3368 _]
              tunnel: w3286 -> [w3363 _]
              tunnel: w3285 -> [w3357 _]
              tunnel: w3266 -> [w3356 _]
              tunnel: w3268 -> [w3341 _]
              tunnel: w3281 -> [w3332 _]
              tunnel: w3265 -> [w3302 _]
              tunnel: w3277 -> [w3309 _]
              tunnel: w3275 -> [w3326 _]
              tunnel: w3274 -> [w3308 _]
              tunnel: w3273 -> [w3317 _]
              tunnel: w3272 -> [w3316 _]
              tunnel: w3271 -> [w3303 _]
              frame No Error {
                n1843 = Index Array(array=w3332, index=w3302) -> (element=w3331:T19)
                n1844 = Unbundle By Name(w3309) -> ("GD LNI old"=w3307:T20)
                n1845 = Index Array(array=w3368, index=w3302) -> (element=w3367:refnum<vi>)
                n1846 = Index Array(array=w3363, index=w3302) -> (element=w3365:refnum<vi>)
                n1847 = Index Array(array=w3326, index=w3302) -> (element=w3325:refnum<vi>)
                n1848 = call "get SPAN active components indices for GD.vi"("error in (no error)"=w3333, "SPAN Idx"=w3302, "SpanInletClusterArray in"=w3332) -> ("error out"=w3345:errorcluster, "aktive Komponenten GD Indices"=w3349:i32[], "SPAN Idx out"=w3350:i32, "SpanInletClusterArray out"=w3351:T19[], "aktive Komponenten Indices additional"=w3337:u16[])  [unwired: 1 in, 3 out]
                n1849 = Unbundle By Name(w3331) -> ("Anzahl Stufen"=w3330:sgl, "Trägergas"=w3328:T26)
                n1850 = call "set Tables Flag from SPANIdx.vi"("SPAN Idx"=w3302) -> ("set Tables"=w3358:bool)  [unwired: 10 in]
                n1851 = call "Index Wertaenderung finden.vi"("neue Tabelle"=w3356, "alte Tabelle"=w3341) -> ("Zeile"=w3354:i32)  [unwired: 7 in, 2 out]
                n1852 = call "Get Gaskomponenten sorted by Concentration.vi"("Fehler (Eingang, kein Fehler)"=w3345, "Component Index"=w3349, "SPAN Idx in (Eingang)"=w3350, "SpanInletClusterArray in (Eingang)"=w3351) -> ("Fehler (Ausgang)"=w3344:errorcluster, "Component Index out"=w3323:i32[], "SPAN Idx out (Ausgang)"=w3327:i32, "SpanInletClusterArray out (Ausgang)"=w3346:T19[], "höchste Konzentration Teilkomponente"=w3310:dbl, "Gesamtkonzentration"=w3311:dbl)  [unwired: 2 in]
                n1853 = Build Array (concatenate)(w3337, w3323) -> (w3342:i32[])
                n1854 = property class="Bool. (strikt)"(reference=w3365, "Value"=FALSE ("Wert")) -> (error out=w3366:errorcluster)  [unwired: 1 in, 1 out]
                n1855 = Index Array(array=w3341, index (row)=w3354, index (col)=0 ("Deaktivierter Index (Spalte)")) -> (element=w3353:string)
                n1856 = Array Size(array=w3342) -> (size(s)=w3348:i32)
                n1857 = Bundle("Zeile"=w3354, w3353) -> (w3352:cluster{"Zeile":i32, string})  [unwired: 1 in]
                n1858 = Bundle("Anzahl Stufen"=w3330, "Trägergas"=w3328, "SPAN Idx out (Ausgang)"=w3327) -> (w3329:T216)  [unwired: 1 in]
                n1859 = call "Get Stufentabellen aller Gaskomponenten.vi"("Fehler (Eingang, kein Fehler)"=w3344, "Component Index"=w3342, "SPAN Idx in (Eingang)"=w3327, "SpanInletClusterArray in (Eingang)"=w3346) -> ("Component Index out"=w3319:i32[], "SPAN Idx out (Ausgang)"=w3321:i32, "SpanInletClusterArray out (Ausgang)"=w3322:T19[], "Stufen Tabelle Array"=w3343:string[][][])  [unwired: 2 in, 2 out]
                n1860 = Bundle(w3308, "GD LNI old"=w3307) -> (w3306:cluster{bool, "GD LNI old":T20})  [unwired: 1 in]
                n1861 = Decrement(x=w3348) -> (x-1=w3347:i32)
                n1862 = Replace Array Subset(array=w3343, new element=w3341, index (dim 0)=w3347) -> (w3335:string[][][])  [unwired: 2 in]
                n1863 = call <vilib>:"Clear Errors.vi"("error in (no error)"=w3366) -> ()  [unwired: 5 in, 2 out]
                n1864 = call "Komponentenauswahl aus SPAN Idx.vi"("Span Iindex"=w3321) -> ("Komponentenauswahl"=w3338:T217)  [unwired: 9 in, 1 out]
                n1865 = for {
                  tunnel: w3358 -> [w3430]
                  tunnel: w3357 -> [w3429]
                  tunnel: [w3428] -> w3339
                  tunnel: w3322 -> [w3426]
                  tunnel: w3321 -> [w3425]
                  tunnel: w3319 -> [w3424] mode=indexing
                  n1866 = call "Komponentenindex aus SPAN.vi"("Component Index in"=w3424, "SPAN Idx in (Eingang)"=w3425, "SpanInletClusterArray in (Eingang)"=w3426) -> ("Komponenten Index"=w3427:u16)  [unwired: 5 in, 3 out]
                  n1867 = case shown="True" w3430 {
                    tunnel: w3427 -> [_ w3433]
                    tunnel: w3429 -> [_ w3432]
                    tunnel: [_ w3431] -> w3428
                    frame False {
                    }
                    frame True {
                      n1868 = call "Stufen abfragen Tabelle vorbereiten.vi"("Komponente in"=w3433, "Tabelle (Eingang)"=w3432) -> ("Fehler (Ausgang)"=w3431:errorcluster)  [unwired: 7 in, 2 out]
                    }
                  }
                }
                n1869 = call "Einzelne Stufe aendern.vi"("Component additional Index"=w3337, "GD-Cluster"=w3329, "Component GD Index"=w3323, "GD LNI Cluster"=w3309, "error in (no error)"=w3339, "Komponentenauswahl"=w3338, "Zeile Punkt Änderung Cluster"=w3352, "Stufen Tabellen in"=w3335) -> ("error out"=w3336:errorcluster, "Component Index out"=w3301:i32, "GD out"=w3340:T218)  [unwired: 1 out]
                n1870 = Array Size(array=w3319) -> (size(s)=w3320:i32)
                n1871 = Array Size(array=w3323) -> (size(s)=w3324:i32)
                n1872 = Decrement(x=w3320) -> (x-1=w3318:i32)
                n1873 = for {
                  tunnel: [w3388] -> w3360
                  tunnel: [w3387] -> w3359
                  tunnel: w3358 -> [w3386]
                  tunnel: w3340 -> [w3385]
                  tunnel: w3322 -> [w3383]
                  tunnel: w3321 -> [w3382]
                  tunnel: w3319 -> [w3381] mode=indexing
                  shift-right: [w3379] -> w3334
                  shift-left: w3336 -> [w3384]
                  tunnel: w3306 -> [w3378]
                  tunnel: w3318 -> [w3377]
                  tunnel: w3317 -> [w3376]
                  tunnel: w3316 -> [w3375]
                  tunnel: w3311 -> [w3374]
                  tunnel: w3310 -> [w3373]
                  i -> [w3380]
                  n1874 = case shown="True" w3386 {
                    tunnel: w3385 -> [w3393 w3416]
                    tunnel: [w3401 w3423] -> w3388
                    tunnel: [w3400 w3422] -> w3387
                    tunnel: w3384 -> [w3399 w3421]
                    tunnel: w3383 -> [w3398 w3420]
                    tunnel: w3382 -> [w3397 w3419]
                    tunnel: w3381 -> [w3396 w3418]
                    tunnel: w3380 -> [w3394 w3413]
                    tunnel: [w3392 w3415] -> w3379
                    tunnel: w3378 -> [_ w3414]
                    tunnel: w3377 -> [_ w3412]
                    tunnel: w3376 -> [_ w3411]
                    tunnel: w3375 -> [_ w3410]
                    tunnel: w3374 -> [_ w3408]
                    tunnel: w3373 -> [_ w3407]
                    frame False {
                      # "nur Stufentabelle\nspeichern"
                      n1875 = call "Komponentenindex aus SPAN.vi"("Component Index in"=w3396, "SPAN Idx in (Eingang)"=w3397, "SpanInletClusterArray in (Eingang)"=w3398) -> ("Component Index out"=w3390:i32, "SPAN Idx out"=w3391:i32, "Komponenten Index"=w3395:u16)  [unwired: 5 in, 1 out]
                      n1876 = Bundle("SPAN Idx out"=w3391, "Component Index out"=w3390) -> (w3389:T219)  [unwired: 1 in]
                      n1877 = call "set Stufentabelle.vi"("Index in"=w3389, "Fehler (Eingang, kein Fehler)"=w3399, "Komponente in"=w3395, "Table Index"=w3394, "GD in"=w3393) -> ("Fehler (Ausgang)"=w3392:errorcluster, "EGAK"=w3400:T26[], "Stufen Tabellen out"=w3401:string[][])  [unwired: 3 in, 1 out]
                    }
                    frame True {
                      # "Ein- Ausgabe\nTabelle schreiben"
